vi "Envia comando serial.vi"(4 "error In":errorcluster, 6 "String a ser Enviado":string, 7 "LNA VISA session (for class)":refnum<visa-resource-name>) -> (0 "error out":errorcluster, 2 "String Enviado":string, 3 "LNA VISA session saida":refnum<visa-resource-name>)   [LabVIEW 2018]
uses:
  <vilib>/Instr/_visa.llb/VISA Flush IO Buffer Mask.ctl
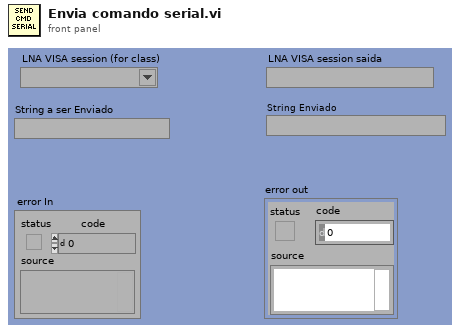
[diagram p1: front panel]
types:
  T1 = typedef "VISA Flush IO Buffer Mask.ctl" = u16
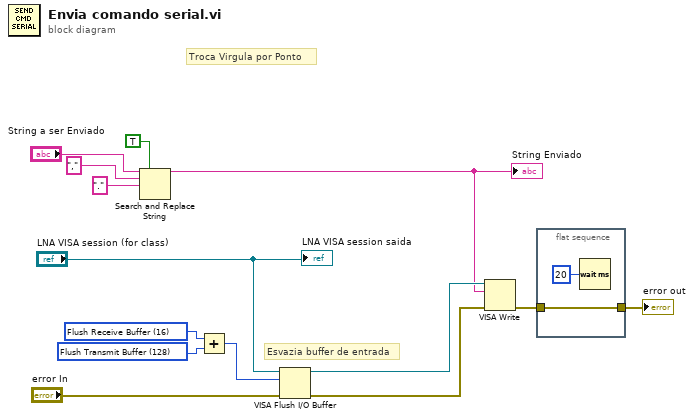
[diagram p0: block diagram]
diagram:
  w4 = T1 128 items=["Flush Receive Buffer"=16, "Write Transmit Buffer to Device"=32, "Flush Receive Buffer (No I/O)"=64, "Flush Transmit Buffer"=128] ("Mask")
  w5 = T1 16 items=["Flush Receive Buffer"=16, "Write Transmit Buffer to Device"=32, "Flush Receive Buffer (No I/O)"=64, "Flush Transmit Buffer"=128] ("Mask")
  # "Esvazia buffer de entrada"
  # "Troca Virgula por Ponto"
  n1 = Search and Replace String(replace all?=TRUE ("replace all? (F)"), input string="String a ser Enviado", search string=",", replace string=".") -> (result string=w6:string)  [unwired: 4 in, 3 out]
  "String Enviado" <- w6
  n2 = Add(x=w5, y=w4) -> (x+y=w3:T1)
  n3 = VISA Flush I/O Buffer(VISA resource name="LNA VISA session (for class)", mask (16)=w3, error in (no error)="error In") -> (VISA resource name out=w12:refnum<visa-resource-name>, error out=w11:errorcluster)
  n4 = VISA Write(VISA resource name=w12, write buffer=w6, error in (no error)=w11) -> (error out=w2:errorcluster)  [unwired: 2 out]
  n5 = flat-sequence {
    tunnel: w2 -> [w16]
    tunnel: [w16] -> w1
    frame #0 {
      n6 = Wait (ms)(milliseconds to wait=u32 20) -> ()  [unwired: 1 out]
    }
  }
  "LNA VISA session saida" <- "LNA VISA session (for class)"
  "error out" <- w1
